vi "Teststand Post Sub Steps STP.vi"(9 "Socket No":u16=1, 10 "STP Data in":T3={"ECU CAN Port"="CAN1", "CMD"=130, "CAN Write Data"=[], "Response Decoder"=enum."String", "String"={"Start Index"=0, "Length"=-1}, "Number"={"MSB Index"=0, "LSB Index"=1}, "Boolean"={"Index"=0, "Bool"={"7"=FALSE, "6"=FALSE, "5"=FALSE, "4"=FALSE, "3"=FALSE, "2"=FALSE, "1"=FALSE, "0"=FALSE, "7 Enabled"=FALSE, "6 Enabled"=FALSE, "5 Enabled"=FALSE, "4 Enabled"=FALSE, "3 Enabled"=FALSE, "2 Enabled"=FALSE, "1 Enabled"=FALSE, "0 Enabled"=FALSE}}} {"CMD" items=["TSW_VERSION(130)"=130, "WAIT_EVENT(132)"=132, "SEQUENCER(133)"=133, "TSW_RESET(150)"=150, "CONFIG_ECU(151)"=151, "TEST_CORE (152)"=152, "TEST_WATCHDOG (153)"=153, "TEST_MONITORING (154)"=154, "READ_MEMORY (162)"=162, "WRITE_ERASE_MEMORY (164)"=164, "COMM_EXTERNAL (190)"=190, "COMM_INTERNAL (195)"=195, "GET_ANALOG_INPUT (210)"=210, "GET_DIGITAL_INPUT (211)"=211, "GET_FREQUENCY_INPUT (212)"=212, "TEST_INPUT_STRUCTURE (214)"=214, "GENERATE_OUTPUT_SIGNAL (220)"=220, "GENERATE_SYNCHRONIZED_OUTPUT_SIGNALS (221)"=221, "eDCU_Specific (250)"=250]; "CAN Write Data" format="%.0x"}, 11 "Sequence Context In":refnum<k7>) -> (0 "error out":errorcluster, 1 "STP Error":T1, 2 "STP Data Out":T2, 3 "Report Text":string)   [LabVIEW 2023, in "LTT_TeststandSteptypes.lvlib"]
uses:
  LTT_TeststandSteptypes.lvlib
  Control/STP Data.ctl
  HardwareAbstractionLayer_LVOOP/CAN/CAN Application Protocols/STP Protocol_class/Ctrls/STP CMD.ctl
  Control/STP Out Data.ctl
  HardwareAbstractionLayer_LVOOP/CAN/CAN Application Protocols/STP Protocol_class/Ctrls/STP Error Cluster.ctl
  HardwareAbstractionLayer_LVOOP/CAN/CAN Application Protocols/STP Protocol_class/Ctrls/STP Input Data.ctl
  HardwareAbstractionLayer_LVOOP/CAN/CAN Application Protocols/STP Protocol_class/STP Protocol.lvclass
panel:
  out "RequestTimeout?":bool
  # "Help : the index will choose the one element in an array and compare its true or false"
  # "Bit"
  # "Value"
  # "Enabled"
  # "Help : if the LSB index is -1 then it will take only MSB value"
  # "Help : if length -1 then it will take the entire array"
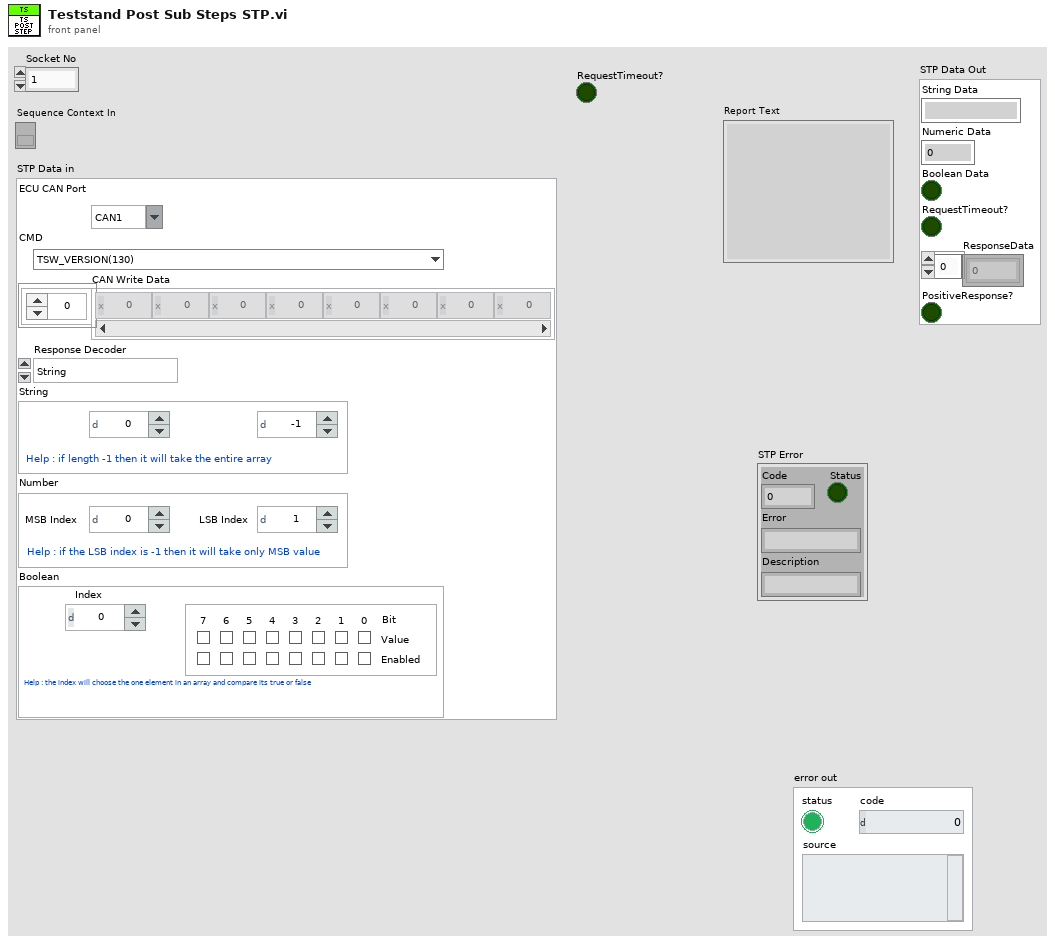
[diagram p1: front panel]
types:
  T1 = typedef "HardwareAbstractionLayer_LVOOP.lvlib/CAN Application Protocols Lib.lvlib/STP Protocol.lvclass/STP Error Cluster.ctl" = cluster{"Status":bool, "Code":u8, "Error":string, "Description":string}
  T2 = typedef "LTT_TeststandSteptypes.lvlib/STP Out Data.ctl" = cluster{"String Data":string, "Numeric Data":dbl, "Boolean Data":bool, "RequestTimeout?":bool, "ResponseData":u8[], "PositiveResponse?":bool}
  T3 = typedef "LTT_TeststandSteptypes.lvlib/STP Data.ctl" = cluster{"ECU CAN Port":string, "CMD":T4, "CAN Write Data":u8[], "Response Decoder":enum16{"String", "Number", "Boolean"}, "String":cluster{"Start Index":i32, "Length":i32}, "Number":cluster{"MSB Index":i32, "LSB Index":i32}, "Boolean":cluster{"Index":i32, "Bool":cluster{"7":bool, "6":bool, "5":bool, "4":bool, "3":bool, "2":bool, "1":bool, "0":bool, "7 Enabled":bool, "6 Enabled":bool, "5 Enabled":bool, "4 Enabled":bool, "3 Enabled":bool, "2 Enabled":bool, "1 Enabled":bool, "0 Enabled":bool}}}
  T4 = typedef "HardwareAbstractionLayer_LVOOP.lvlib/CAN Application Protocols Lib.lvlib/STP Protocol.lvclass/STP CMD.ctl" = u8
  T5 = typedef "HardwareAbstractionLayer_LVOOP.lvlib/CAN Application Protocols Lib.lvlib/STP Protocol.lvclass/STP Input Data.ctl" = cluster{"TxID":u32, "RxID":u32, "CMD":T4, "RQ Data":u8[], "+veResponseCode":u8, "ResponseTimeout (S)":dbl}
  T6 = typedef "HardwareAbstractionLayer_LVOOP.lvlib/CAN HAL Lib.lvlib/CAN.lvclass/CAN Init Ctrl.ctl" = cluster{"XNET Interface":refnum<k21>, "Baud Rate":u64, "CAN:Termination":u32, "Echo Transmit?":bool, "scope (normal)":T7}
  T7 = typedef "XNET Control Scope.ctl" = u32
  T8 = cluster{"Refnum out":refnum<k21>, "CAN Init Data":T6, "CAN_RxID":u32, "CAN_TxID":u32, "Timeout":dbl}
  T9 = typedef "HardwareAbstractionLayer_LVOOP.lvlib/CAN Application Protocols Lib.lvlib/STP Protocol.lvclass/STP Output Data.ctl" = cluster{"ResponseData":u8[], "ResponseData(ASCII)":string, "PositiveResponse?":bool, "STP Error":T1}
  T10 = cluster{"7":bool, "6":bool, "5":bool, "4":bool, "3":bool, "2":bool, "1":bool, "0":bool, "7 Enabled":bool, "6 Enabled":bool, "5 Enabled":bool, "4 Enabled":bool, "3 Enabled":bool, "2 Enabled":bool, "1 Enabled":bool, "0 Enabled":bool}
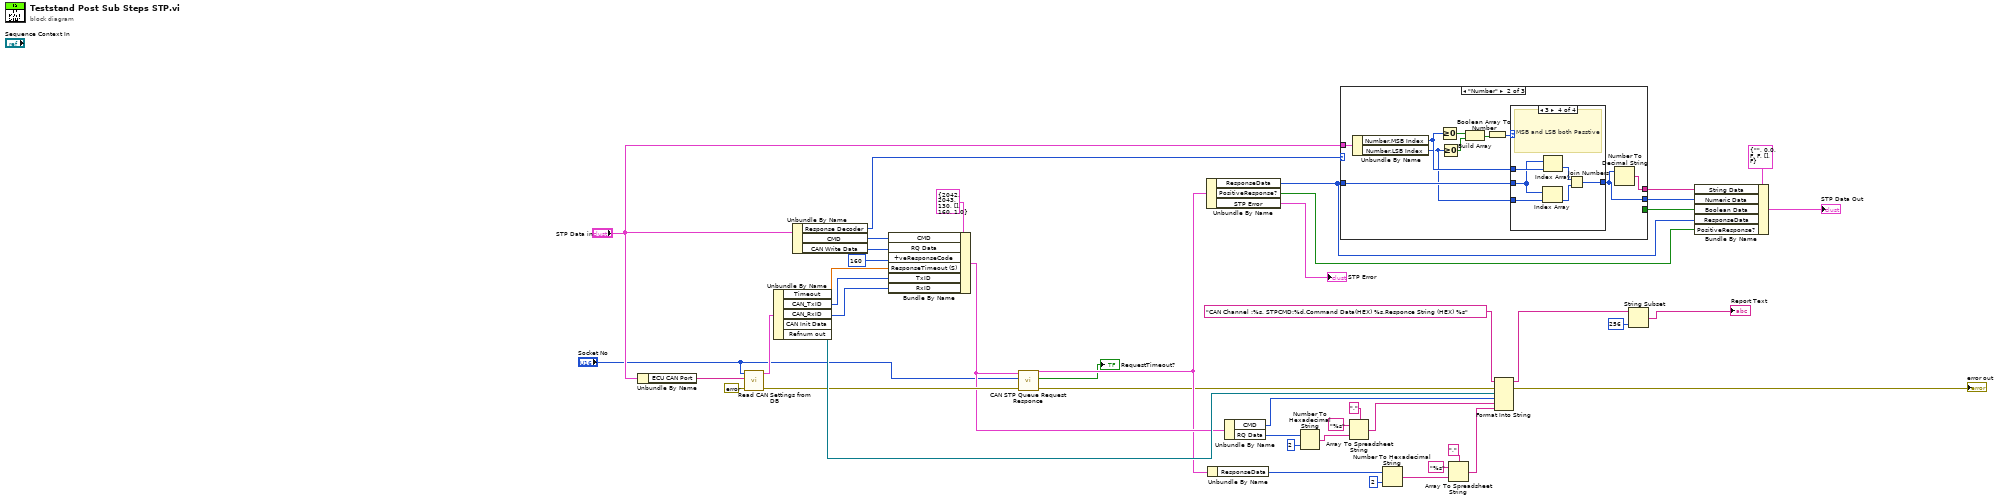
[diagram p0: block diagram]
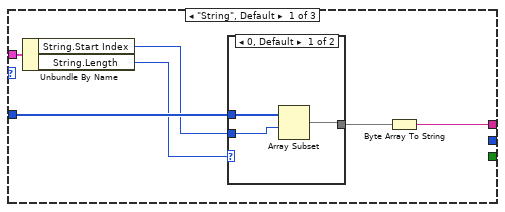
[diagram p2: hidden frame]
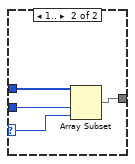
[diagram p3: hidden frame]
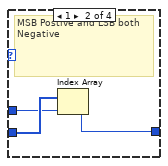
[diagram p5: hidden frame]
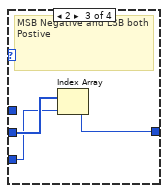
[diagram p6: hidden frame]
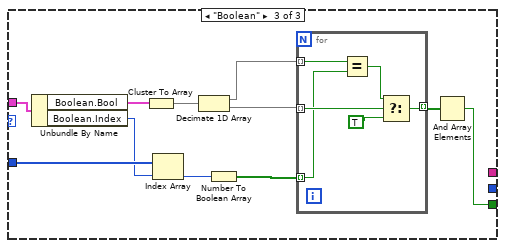
[diagram p7: hidden frame]
diagram:
  n1 = Unbundle By Name("STP Data in") -> ("ECU CAN Port"=w12:string)
  n2 = call "Read CAN Settings from DB.vi"("error in"=errorcluster {"status"=FALSE, "code"=0, "source"=""}, "ECU CAN Port"=w12, "Socket No"="Socket No") -> ("error out"=w6:errorcluster, "Read CAN Setting"=w11:T8)  [unwired: 7 in]
  n3 = Unbundle By Name(w11) -> ("Timeout"=w10:dbl, "CAN_TxID"=w9:u32, "CAN_RxID"=w8:u32, "Refnum out"=w7:refnum<k21>)  [unwired: 1 out]
  n4 = Unbundle By Name("STP Data in") -> ("Response Decoder"=w31:enum16{"String", "Number", "Boolean"}, "CMD"=w44:T4, "CAN Write Data"=w43:u8[])
  n5 = Bundle By Name(cluster=T5 {"TxID"=2042, "RxID"=2043, "CMD"=130, "RQ Data"=[], "+veResponseCode"=160, "ResponseTimeout (S)"=1.0} ("STP Input Data"), "CMD"=w44, "RQ Data"=w43, "+veResponseCode"=u8 160, "ResponseTimeout (S)"=w10, "TxID"=w9, "RxID"=w8) -> (w5:T5)
  n6 = call "CAN STP Queue Request Responce.vi"("error in (no error)"=w6, "Socket No"="Socket No", "STP Input Data"=w5) -> ("error out"=w1:errorcluster, "RequestTimeout?"=→"RequestTimeout?":bool, "STP Output Data"=w3:T9)  [unwired: 6 in]
  n7 = Unbundle By Name(w3) -> ("ResponseData"=w36:u8[], "PositiveResponse?"=w34:bool, "STP Error"=→"STP Error":T1)
  n8 = Unbundle By Name(w3) -> ("ResponseData"=w19:u8[])
  n9 = Unbundle By Name(w5) -> ("CMD"=w30:T4, "RQ Data"=w21:u8[])
  n10 = Number To Hexadecimal String(1:i16 2 ("width (-)"), 2:w21) -> (0:w25:string[])
  n11 = case shown="\"Number\"" w31 {
    tunnel: w36 -> [w50 w63 w88]
    tunnel: "STP Data in" -> [w51 w68 w91]
    tunnel: [w46 w59 _] -> w39
    tunnel: [_ w60 _] -> w38
    tunnel: [_ _ w81] -> w37
    frame "String", Default {
      n12 = Unbundle By Name(w51) -> ("String.Start Index"=w49:i32, "String.Length"=w48:i32)
      n13 = case shown="0, Default" w48 {
        selector: w48 -> [_ w56]
        tunnel: w50 -> [w54 w58]
        tunnel: w49 -> [w53 w57]
        tunnel: [w52 w55] -> w47
        frame 0, Default {
          n14 = Array Subset(array=w54, index=w53) -> (w52:u8[])  [unwired: 1 in]
        }
        frame 1.. {
          n15 = Array Subset(array=w58, index=w57, length=w56) -> (w55:u8[])
        }
      }
      n16 = Byte Array To String(unsigned byte array=w47) -> (string=w46:string)
    }
    frame "Number" {
      n17 = Unbundle By Name(w68) -> ("Number.MSB Index"=w62:i32, "Number.LSB Index"=w61:i32)
      n18 = Greater Or Equal To 0?(x=w62) -> (x >= 0?=w67:bool)
      n19 = Greater Or Equal To 0?(x=w61) -> (x >= 0?=w66:bool)
      n20 = Build Array(w67, w66) -> (w65:bool[])
      n21 = Boolean Array To Number(Boolean array=w65) -> (number=w64:u32)
      n22 = case shown="3" w64 {
        tunnel: w63 -> [_ w71 w74 w79]
        tunnel: w62 -> [_ w70 _ w80]
        tunnel: w61 -> [_ _ w72 w78]
        tunnel: [_ w69 w73 w75] -> w60
        frame 0, Default {
          # "MSB and LSB both Negative"
        }
        frame 1 {
          # "MSB Postive and LSB both Negative"
          n23 = Index Array(array=w71, index=w70) -> (element=w69:u8)
        }
        frame 2 {
          # "MSB Negative and LSB both Postive"
          n24 = Index Array(array=w74, index=w72) -> (element=w73:u8)
        }
        frame 3 {
          # "MSB and LSB both Passtive"
          n25 = Index Array(array=w79, index=w78) -> (element=w76:u8)
          n26 = Index Array(array=w79, index=w80) -> (element=w77:u8)
          n27 = Join Numbers(hi=w77, lo=w76) -> ((hi.lo)=w75:u16)
        }
      }
      n28 = Number To Decimal String(number=w60) -> (decimal integer string=w59:string)  [unwired: 1 in]
    }
    frame "Boolean" {
      n29 = Unbundle By Name(w91) -> ("Boolean.Bool"=w90:T10, "Boolean.Index"=w87:i32)
      n30 = Cluster To Array(cluster=w90) -> (array=w89:bool[])
      n31 = Index Array(array=w88, index=w87) -> (element=w86:u8)
      n32 = Decimate 1D Array(w89) -> (w84:bool[], w83:bool[])
      n33 = Number To Boolean Array(number=w86) -> (Boolean array=w85:bool[])
      n34 = for {
        tunnel: w85 -> [w95] mode=indexing
        tunnel: w84 -> [w96] mode=indexing
        tunnel: w83 -> [w97] mode=indexing
        tunnel: [w92] -> w82 mode=indexing
        n35 = Equal?(x=w96, y=w95) -> (x = y?=w94:bool)
        n36 = Select(t=w94, s=w97, f=TRUE) -> (s? t:f=w92:bool)
      }
      n37 = And Array Elements(Boolean array=w82) -> (logical AND=w81:bool)
    }
  }
  n38 = Array To Spreadsheet String(delimiter (Tab)=",", array=w25, 3:"%s" ("format string")) -> (spreadsheet string=w28:string)
  n39 = Number To Hexadecimal String(1:i16 2 ("width (-)"), 2:w19) -> (0:w18:string[])
  n40 = Array To Spreadsheet String(delimiter (Tab)=",", array=w18, 3:"%s" ("format string")) -> (spreadsheet string=w17:string)
  n41 = Format Into String(format string="CAN Channel :%s, STPCMD:%d,Command Data(HEX) %s,Responce String (HEX) %s", error in=w1, w7, w30, w28, w17) -> (resulting string=w16:string, error out=→"error out":errorcluster)  [unwired: 1 in]
  n42 = String Subset(string=w16, length (rest)=256 ("length (rest)")) -> (substring=→"Report Text":string)  [unwired: 1 in]
  n43 = Bundle By Name(cluster=T2 {"String Data"="", "Numeric Data"=0.0, "Boolean Data"=FALSE, "RequestTimeout?"=FALSE, "ResponseData"=[], "PositiveResponse?"=FALSE} ("STP Data Out"), "String Data"=w39, "Numeric Data"=w38, "Boolean Data"=w37, "ResponseData"=w36, "PositiveResponse?"=w34) -> (→"STP Data Out":T2)
